vi "ADXL345 I2C Read XY.vi"(8 "error in":errorcluster, 11 "I2CDevRef":T1 {"Device Address" format="%.0x"}) -> (0 "error out":errorcluster, 2 "Acceleration XY":dbl[](array[numeric]), 3 "I2CDevRef Out":T1 {"Device Address" format="%.0x"})   [LabVIEW 2013]
uses:
  <vilib>/Rock Robotics/WPI/I2C/WPI_I2CDevRef.ctl
  <vilib>/Rock Robotics/SystemInterfaces/Typedef/FPGA_TypedefDigitalModule.ctl
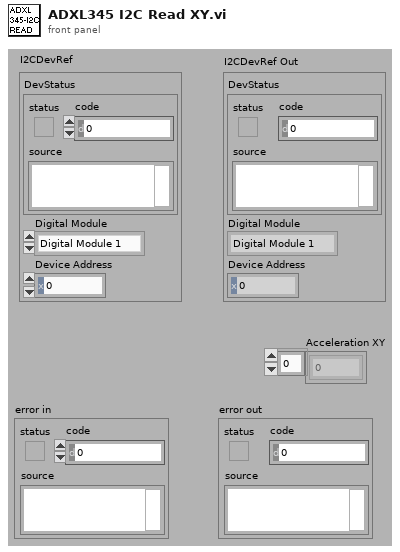
[diagram p1: front panel]
types:
  T1 = typedef "WPI_I2CDevRef.ctl" = cluster{"DevStatus":errorcluster, "Digital Module":T2, "Device Address":u8}
  T2 = typedef "FPGA_TypedefDigitalModule.ctl" = enum16{"Digital Module 1", "Digital Module 2"}
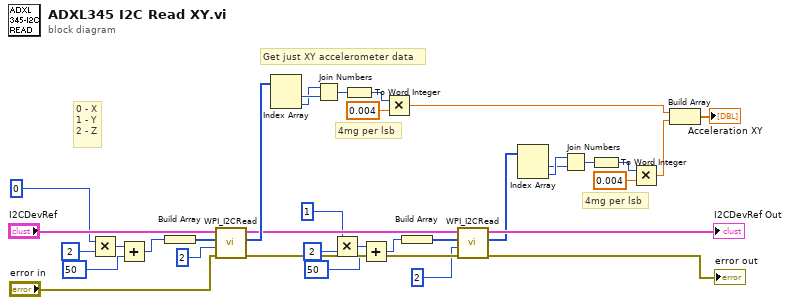
[diagram p0: block diagram]
diagram:
  # "Get just XY accelerometer data"
  # "4mg per lsb"
  # "0 - X\n1 - Y\n2 - Z"
  # "4mg per lsb"
  n1 = Multiply(x=u8 0, y=u8 2 ("Data To Send")) -> (x*y=w35:u8)
  n2 = Add(x=w35, y=u8 50 ("Data To Send")) -> (x+y=w25:u8)
  n3 = Build Array(w25) -> (w24:u8[])
  n4 = call <vilib>:"WPI_I2CRead.vi"("error in (no error)"="error in", "I2CBytesToRead"=u8 2, "I2CRegister"=w24, "I2CDevRef"="I2CDevRef") -> ("error out"=w19:errorcluster, "Data Out"=w29:u8[], "I2CDevRef"=w20:T1)  [unwired: 1 in, 4 out]
  n5 = Index Array(array=w29) -> (element #1=w27:u8, element #2=w26:u8)  [unwired: 2 in]
  n6 = Join Numbers(hi=w26, lo=w27) -> ((hi.lo)=w28:u16)
  n7 = Multiply(x=u8 1, y=u8 2 ("Data To Send")) -> (x*y=w16:u8)
  n8 = To Word Integer(number=w28) -> (16bit integer=w22:i16)
  n9 = Add(x=w16, y=u8 50 ("Data To Send")) -> (x+y=w13:u8)
  n10 = Multiply(x=w22, y=0.004) -> (x*y=w2:dbl)
  n11 = Build Array(w13) -> (w11:u8[])
  n12 = call <vilib>:"WPI_I2CRead.vi"("error in (no error)"=w19, "I2CBytesToRead"=u8 2, "I2CRegister"=w11, "I2CDevRef"=w20) -> ("error out"=→"error out":errorcluster, "Data Out"=w4:u8[], "I2CDevRef"=→"I2CDevRef Out":T1)  [unwired: 1 in, 4 out]
  n13 = Index Array(array=w4) -> (element #1=w7:u8, element #2=w8:u8)  [unwired: 2 in]
  n14 = Join Numbers(hi=w8, lo=w7) -> ((hi.lo)=w6:u16)
  n15 = To Word Integer(number=w6) -> (16bit integer=w9:i16)
  n16 = Multiply(x=w9, y=0.004) -> (x*y=w3:dbl)
  n17 = Build Array(w2, w3) -> (→"Acceleration XY":dbl[])
